vi "Popualte Names Init.vi"(8 "error in (no error)":errorcluster, 10 "Engine Name":string, 11 "Destination Path":path) -> (0 "error out":errorcluster, 2 "Communication FIFOs Elements":refnum<vi>[](array[refnum]), 3 "Communication FIFOs Refnum":refnum<vi>)   [LabVIEW 2014, in "Initialization and IO Node Scripting.lvlib"]
uses:
  Initialization and IO Node Scripting.lvlib
  <vilib>/Utility/traverseref.llb/TRef TravTarget.ctl
  <vilib>/Utility/traverseref.llb/VI Scripting - Traverse.lvlib
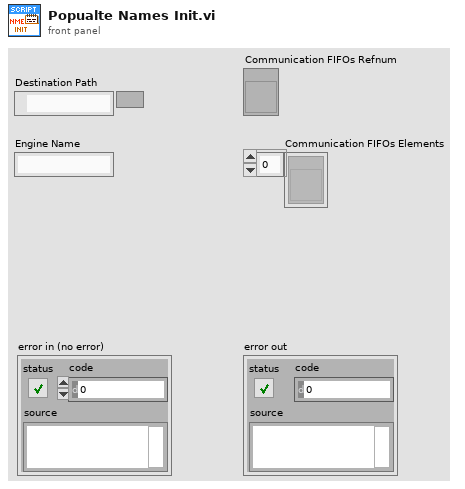
[diagram p1: front panel]
types:
  T1 = typedef "TRef TravTarget.ctl" = enum16{"FP", "BD", "Other"}
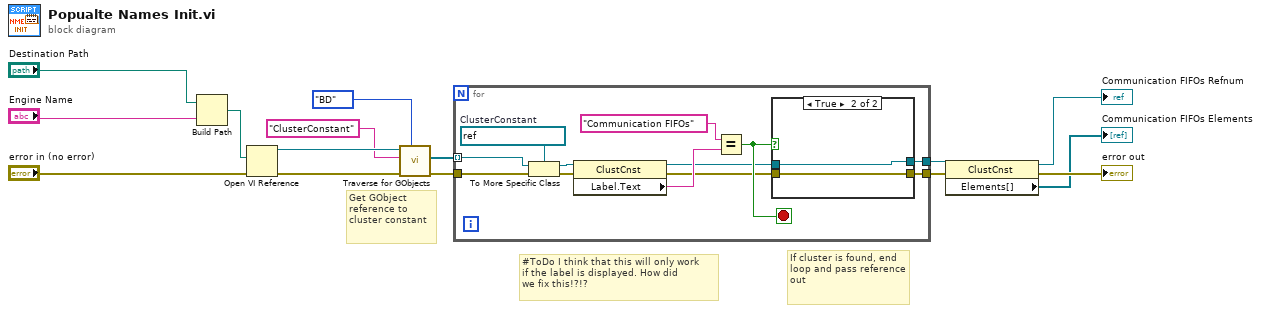
[diagram p0: block diagram]
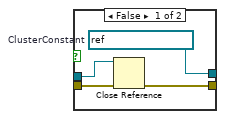
[diagram p2: hidden frame]
diagram:
  # "#ToDo I think that this will only work\nif the label is displayed. How did\nwe fix this!?!?"
  # "If cluster is found, end loop and pass reference out"
  # "Get GObject reference to cluster constant"
  n1 = Build Path(base path="Destination Path", name or relative path="Engine Name") -> (appended path=w8:path)
  n2 = Open VI Reference(vi path=w8, error in (no error)="error in (no error)") -> (vi reference=w11:refnum<vi>, error out=w12:errorcluster)  [unwired: 4 in]
  n3 = call <vilib>:"Traverse for GObjects.vi"("Traverse Target"=TRef_TravTarget."BD", "error in (no error)"=w12, "Class Name"="ClusterConstant", "VI Refnum"=w11) -> ("error out"=w14:errorcluster, "References"=w13:refnum<vi>[])  [unwired: 4 in, 2 out]
  n4 = for {
    tunnel: w13 -> [w25] mode=indexing
    tunnel: w14 -> [w26]
    tunnel: [w17] -> w6
    tunnel: [w16] -> w7
    stop <- w20 stop-if-true
    w27 = refnum<vi> refnum  # ClusterConstant
    n5 = To More Specific Class(target class=w27, reference=w25, error in=w26) -> (specific class reference=w23:refnum<vi>, error out=w24:errorcluster)
    n6 = property class="ClustCnst"(reference=w23, error in=w24) -> (reference out=w18:refnum<vi>, error out=w19:errorcluster, "Label.Text"=w22:string)
    n7 = Equal?(x="Communication FIFOs", y=w22) -> (x = y?=w20:bool)
    n8 = case shown="True" w20 {
      tunnel: w19 -> [w31 w33]
      tunnel: w18 -> [w30 w32]
      tunnel: [w28 w33] -> w16
      tunnel: [w29 w32] -> w17
      frame False {
        w29 = refnum<vi> refnum  # ClusterConstant
        n9 = Close Reference(reference=w30, error in (no error)=w31) -> (error out=w28:errorcluster)
      }
      frame True {
      }
    }
  }
  n10 = property class="ClustCnst"(reference=w6, error in=w7) -> (reference out=→"Communication FIFOs Refnum":refnum<vi>, error out=→"error out":errorcluster, "Elements[]"=→"Communication FIFOs Elements":refnum<vi>[])
